vi "List of Variables.vi"(1 "Table":i32[][](array[numeric])) -> (0 "List of variables":i32[](array[numeric]))   [LabVIEW 2017, in "NI_Gmath.lvlib"]
uses:
  <vilib>/gmath/NI_Gmath.lvlib
panel:
  # "operator"
  # "register1"
  # "register2"
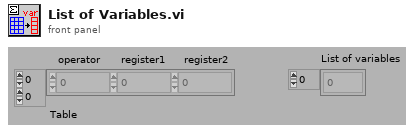
[diagram p1: front panel]
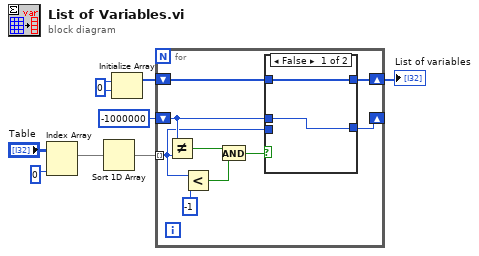
[diagram p0: block diagram]
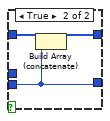
[diagram p2: hidden frame]
diagram:
  w6 = 0
  n1 = Index Array(array="Table", index (col)=0) -> (element=w2:i32[])  [unwired: 1 in]
  n2 = Sort 1D Array(array=w2) -> (sorted array=w1:i32[])
  n3 = Initialize Array(w6, w6) -> (w5:i32[])
  n4 = for {
    shift-right: [w15] -> _
    shift-left: -1000000 -> [w14]
    tunnel: w1 -> [w13] mode=indexing
    shift-right: [w16] -> w3
    shift-left: w5 -> [w17]
    n5 = Not Equal?(x=w14, y=w13) -> (x != y?=w11:bool)
    n6 = Less?(x=w13, y=-1) -> (x < y?=w10:bool)
    n7 = And(x=w11, y=w10) -> (x .and. y?=w9:bool)
    n8 = case shown="False" w9 {
      tunnel: w17 -> [w19 w22]
      tunnel: [w19 w21] -> w16
      tunnel: w13 -> [_ w20]
      tunnel: [w18 w20] -> w15
      tunnel: w14 -> [w18 _]
      frame False {
      }
      frame True {
        n9 = Build Array (concatenate)(w22, w20) -> (w21:i32[])
      }
    }
  }
  "List of variables" <- w3
